vi "Piece Polynomial Function Approx and Comp.vi"() -> ()   [LabVIEW 2023]
doc: "This example shows how to use wavelets to approximate the piece polynomial function. When the order is high enough, the wavelet transform generates only high-amplitude coefficients at discontinuous points. Most of the coefficients at continuous points are close to zero. For this reason, wavelets are widely applied in signal compression. This example uses the WA Discrete Wavelet Transform VI and the WA Inverse Discrete Wavelet Transform VI.\n\n<b>Instructions:</b>\n1) Run this VI.\n2) Change the <b>Wavelet</b> type and <b>Levels</b>.\n3) Browse the Block Diagram of this example to learn how to use wavelets to approximate the piece polynomial function."
uses:
  <vilib>/addons/Wavelet Analysis/typedefs.llb/WA Data.ctl
  <vilib>/addons/Wavelet Analysis/discrete wavelet transform.llb/WA 1D Discrete Wavelet Transform (Waveform).vi
  <vilib>/addons/Wavelet Analysis/discrete wavelet transform.llb/WA Inverse 1D Discrete Wavelet Transform (Waveform).vi
  <vilib>/addons/_Advanced Signal Processing/NI_AdvSigProcWA.lvlib
panel:
  out "Signal":waveform(dbl)(graph)
  out "Coefficients\nless than 0.1":dbl format="%#.1f %"
  out "DWT Coefficients":waveform(dbl)(graph)
  out "Reconstructed Signal":waveform(dbl)(graph)
  in  "Wavelet":u16(ring) items=["db02"=0, "db03"=1, "db04"=2, "db05"=3, "db06"=4, "db07"=5, "db08"=6, "db09"=7, "db10"=8, "db11"=9, "db12"=10, "db13"=11, "db14"=12, "Haar"=13, "bior1_3"=14, "bior1_5"=15, "bior2_2"=16, "bior2_4"=17, "bior2_6"=18, "bior2_8"=19, "bior3_1"=20, "bior3_3"=21, "bior3_5"=22, "bior3_7"=23, "bior3_9"=24, "bior4_4 (FBI)"=25, "bior5_5"=38, "bior6_8"=39, "coif1"=26, "coif2"=27, "coif3"=28, "coif4"=29, "coif5"=30, "sym2"=31, "sym3"=32, "sym4"=33, "sym5"=34, "sym6"=35, "sym7"=36, "sym8"=37]
  in  "Levels":i32=10
  # "Overview: Shows how to use wavelets to approximate the piece polynomial function. \nRequirements: LabVIEW Full Development System, Advanced Signal Processing Toolkit\nInstructions: \n1. Run this VI.\n2. Change the Wavelet type and Levels.\n3. Browse the block diagram of this example to learn how to use wavelets to approximate the piece polynomial function."
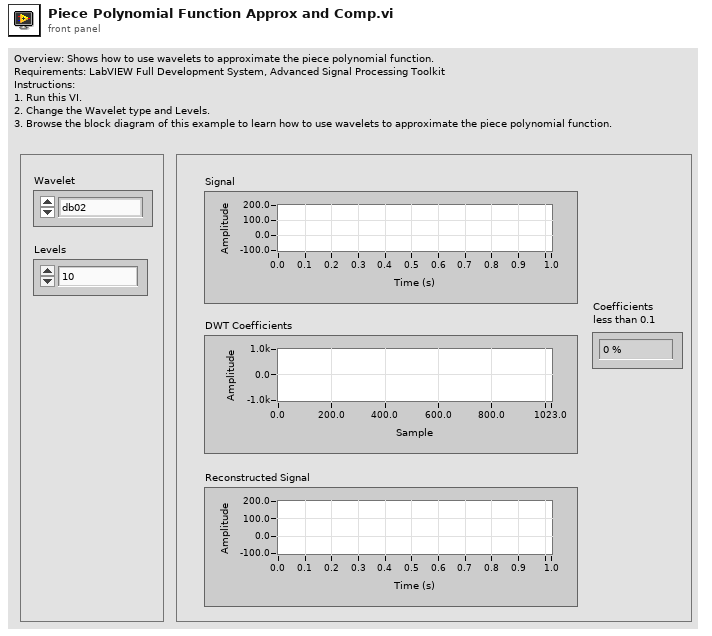
[diagram p1: front panel]
types:
  T1 = typedef "NI_AdvSigProcWA.lvlib/WA Data.ctl" = u16
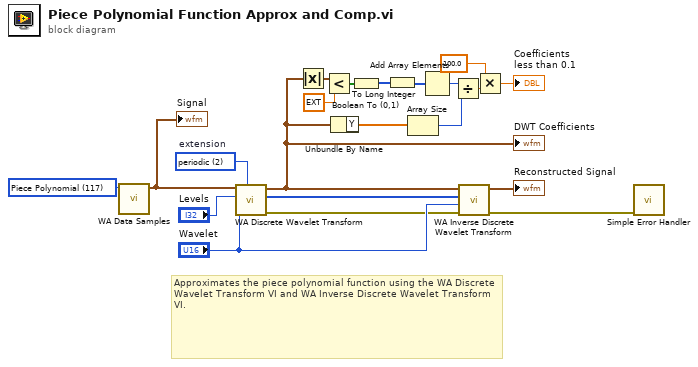
[diagram p0: block diagram]
diagram:
  w5 = T1 117 items=["1D Example Data"=100, "-"=101, "Doppler"=102, "HOP"=103, "TF Sine"=104, "Noisy Doppler"=105, "Sea Temperature"=106, "Sp500"=107, "Power Line"=108, "Engine Knocking"=109, "HeaviSine"=110, "Bumps"=111, "Blocks"=112, "Piece Regular"=113, "HypChirps"=114, "LinChirps"=115, "Chirps"=116, "Piece Polynomial"=117, "ECG"=131, "-"=118, "2D Example Data"=119, "-"=120, "Finger Print (Image)"=121, "Iris Flower (Image)"=122, "Mammogram (Image)"=123, "Lake (Image)"=127, "Two Can 1 (Image)"=132, "Two Can 2 (Image)"=133, "Camera Man (Image)"=134] ("data")
  w18 = u16 2 items=["zero padding", "symmetric", "periodic", "spline"]  # extension
  # "Approximates the piece polynomial function using the WA Discrete Wavelet Transform VI and WA Inverse Discrete Wavelet Transform VI."
  n1 = call <vilib>:"WA Data Samples.vi"("data"=w5) -> ("signal"=w9:waveform(dbl))  [unwired: 10 out]
  "Signal" <- w9
  n2 = call-poly <vilib>:"WA Discrete Wavelet Transform.vi"("extension"=w18, "wavelet"="Wavelet", "levels"="Levels", "signal"=w9) -> ("error out"=w4:errorcluster, "length"=w20:i32[], "DWT coef"=w8:waveform(dbl))  [unwired: 1 in, 4 out]
  "DWT Coefficients" <- w8
  n3 = Absolute Value(x=w8) -> (abs(x)=w17:waveform(dbl))
  n4 = Less?(x=w17, y=ext 0.1) -> (x < y?=w16:bool[])
  n5 = Unbundle By Name(w8) -> ("Y"=w7:dbl[])
  n6 = Boolean To (0,1)(Boolean=w16) -> (0, 1=w2:i16[])
  n7 = To Long Integer(number=w2) -> (32bit integer=w1:i32[])
  n8 = Array Size(array=w7) -> (size(s)=w6:i32)
  n9 = Add Array Elements(numeric array=w1) -> (sum=w15:i32)
  n10 = Divide(x=w15, y=w6) -> (x/y=w14:dbl)
  n11 = call-poly <vilib>:"WA Inverse Discrete Wavelet Transform.vi"("error in (no error)"=w4, "wavelet"="Wavelet", "length"=w20, "DWT coef"=w8) -> ("error out"=w3:errorcluster, "signal"=→"Reconstructed Signal":waveform(dbl))  [unwired: 6 out]
  n12 = Multiply(x=100.0, y=w14) -> (x*y=→"Coefficients\nless than 0.1":dbl)
  n13 = call <vilib>:"Simple Error Handler.vi"("error in (no error)"=w3) -> ()  [unwired: 4 in, 5 out]
